vi "nanocal -- nuclear schottky fit V3.vi"() -> ()   [LabVIEW 2020] (continued)
-> 45.000000000000  |>   , \r80135 ->   <| \"ζ\"->  0.000000000000  , \"τ1\"-> 0.000000000000  , \"τS\"-> 0.000000000000  , \"τN\"-> 0.000000000000  , \"τC\"-> 0.000000000000  , \"κ0\"-> 0.000000000000  , \"mm1\"-> 0.000000000000  , \"mm2\"-> 0.000000000000  , \"mm3\"-> 0.000000000000  , \"T\"->  0.830000000000  , \"B\"-> 12.000000000000  , \"θ\"-> 45.000000000000  |>   , \r80136 ->   <| \"ζ\"->  0.000000000000  , \"τ1\"-> 0.000000000000  , \"τS\"-> 0.000000000000  , \"τN\"-> 0.000000000000  , \"τC\"-> 0.000000000000  , \"κ0\"-> 0.000000000000  , \"mm1\"-> 0.000000000000  , \"mm2\"-> 0.000000000000  , \"mm3\"-> 0.000000000000  , \"T\"->  1.130000000000  , \"B\"-> 12.000000000000  , \"θ\"-> 45.000000000000  |>   , \r80137 ->   <| \"ζ\"->  0.000000000000  , \"τ1\"-> 0.000000000000  , \"τS\"-> 0.000000000000  , \"τN\"-> 0.000000000000  , \"τC\"-> 0.000000000000  , \"κ0\"-> 0.000000000000  , \"mm1\"-> 0.000000000000  , \"mm2\"-> 0.000000000000  , \"mm3\"-> 0.000000000000  , \"T\"->  1.900000000000  , \"B\"-> 12.000000000000  , \"θ\"-> 45.000000000000  |>   , \r80138 ->   <| \"ζ\"->  0.000000000000  , \"τ1\"-> 0.000000000000  , \"τS\"-> 0.000000000000  , \"τN\"-> 0.000000000000  , \"τC\"-> 0.000000000000  , \"κ0\"-> 0.000000000000  , \"mm1\"-> 0.000000000000  , \"mm2\"-> 0.000000000000  , \"mm3\"-> 0.000000000000  , \"T\"->  3.100000000000  , \"B\"-> 12.000000000000  , \"θ\"-> 45.000000000000  |>   , \r80139 ->   <| \"ζ\"->  0.000000000000  , \"τ1\"-> 0.000000000000  , \"τS\"-> 0.000000000000  , \"τN\"-> 0.000000000000  , \"τC\"-> 0.000000000000  , \"κ0\"-> 0.000000000000  , \"mm1\"-> 0.000000000000  , \"mm2\"-> 0.000000000000  , \"mm3\"-> 0.000000000000  , \"T\"->  5.700000000000  , \"B\"-> 12.000000000000  , \"θ\"-> 45.000000000000  |>   , \r"
  out "string OUT":string="  4026 ->   <| \"ζ\"->  0.380655948508  , \"τ1\"-> 0.067955996733  , \"τS\"-> 0.077431477619  , \"τN\"-> 0.380655948508  , \"τC\"-> 0.001948284419  , \"κ0\"-> 0.000000000405  , \"mm1\"-> 0.000000000000  , \"mm2\"-> 0.000000000000  , \"mm3\"-> 0.000000000000  , \"T\"->  0.127000000000  , \"B\"-> 12.000000000000  , \"θ\"-> 60.000000000000  |>   , \r4027 ->   <| \"ζ\"->  0.301371774455  , \"τ1\"-> 0.068371484218  , \"τS\"-> 0.061790748646  , \"τN\"-> 0.216325501043  , \"τC\"-> 0.002093631430  , \"κ0\"-> 0.000000000652  , \"mm1\"-> 0.000000000000  , \"mm2\"-> 0.000000000000  , \"mm3\"-> 0.000000000000  , \"T\"->  0.150000000000  , \"B\"-> 12.000000000000  , \"θ\"-> 60.000000000000  |>   , \r4028 ->   <| \"ζ\"->  0.246466162800  , \"τ1\"-> 0.063598094006  , \"τS\"-> 0.040287819160  , \"τN\"-> 0.158425596558  , \"τC\"-> 0.002271690953  , \"κ0\"-> 0.000000000764  , \"mm1\"-> 0.000000000000  , \"mm2\"-> 0.000000000000  , \"mm3\"-> 0.000000000000  , \"T\"->  0.179000000000  , \"B\"-> 12.000000000000  , \"θ\"-> 60.000000000000  |>   , \r4029 ->   <| \"ζ\"->  0.189727451301  , \"τ1\"-> 0.058299219384  , \"τS\"-> 0.037057198532  , \"τN\"-> 0.081832461227  , \"τC\"-> 0.002345641238  , \"κ0\"-> 0.000000001055  , \"mm1\"-> 0.000000000000  , \"mm2\"-> 0.000000000000  , \"mm3\"-> 0.000000000000  , \"T\"->  0.200000000000  , \"B\"-> 12.000000000000  , \"θ\"-> 60.000000000000  |>   , \r4030 ->   <| \"ζ\"->  0.139910467625  , \"τ1\"-> 0.047050769060  , \"τS\"-> 0.031171501064  , \"τN\"-> 0.041998910400  , \"τC\"-> 0.002916001976  , \"κ0\"-> 0.000000001342  , \"mm1\"-> 0.000000000000  , \"mm2\"-> 0.000000000000  , \"mm3\"-> 0.000000000000  , \"T\"->  0.240000000000  , \"B\"-> 12.000000000000  , \"θ\"-> 60.000000000000  |>   , \r4031 ->   <| \"ζ\"->  0.099227356109  , \"τ1\"-> 0.042371773796  , \"τS\"-> 0.026407434530  , \"τN\"-> 0.023302306750  , \"τC\"-> 0.003363353135  , \"κ0\"-> 0.000000001685  , \"mm1\"-> 0.000000000000  , \"mm2\"-> 0.000000000000  , \"mm3\"-> 0.000000000000  , \"T\"->  0.287000000000  , \"B\"-> 12.000000000000  , \"θ\"-> 60.000000000000  |>   , \r4032 ->   <| \"ζ\"->  0.076929995365  , \"τ1\"-> 0.033595523097  , \"τS\"-> 0.023151959369  , \"τN\"-> 0.012952644411  , \"τC\"-> 0.004200734342  , \"κ0\"-> 0.000000002024  , \"mm1\"-> 0.000000000000  , \"mm2\"-> 0.000000000000  , \"mm3\"-> 0.000000000000  , \"T\"->  0.330000000000  , \"B\"-> 12.000000000000  , \"θ\"-> 60.000000000000  |>   , \r4033 ->   <| \"ζ\"->  0.051029693776  , \"τ1\"-> 0.027044732579  , \"τS\"-> 0.020325597844  , \"τN\"-> 0.004901643856  , \"τC\"-> 0.005324185887  , \"κ0\"-> 0.000000002659  , \"mm1\"-> 0.000000000000  , \"mm2\"-> 0.000000000000  , \"mm3\"-> 0.000000000000  , \"T\"->  0.430000000000  , \"B\"-> 12.000000000000  , \"θ\"-> 60.000000000000  |>   , \r4034 ->   <| \"ζ\"->  0.041895708972  , \"τ1\"-> 0.024266785024  , \"τS\"-> 0.017749465045  , \"τN\"-> 0.003280175510  , \"τC\"-> 0.006877927658  , \"κ0\"-> 0.000000003199  , \"mm1\"-> 0.000000000000  , \"mm2\"-> 0.000000000000  , \"mm3\"-> 0.000000000000  , \"T\"->  0.510000000000  , \"B\"-> 12.000000000000  , \"θ\"-> 60.000000000000  |>   , \r4035 ->   <| \"ζ\"->  0.038450971441  , \"τ1\"-> 0.022519642738  , \"τS\"-> 0.015666742742  , \"τN\"-> 0.001856597287  , \"τC\"-> 0.008327032616  , \"κ0\"-> 0.000000003902  , \"mm1\"-> 0.000000000000  , \"mm2\"-> 0.000000000000  , \"mm3\"-> 0.000000000000  , \"T\"->  0.620000000000  , \"B\"-> 12.000000000000  , \"θ\"-> 60.000000000000  |>   , \r4036 ->   <| \"ζ\"->  0.030292839572  , \"τ1\"-> 0.021747519944  , \"τS\"-> 0.012455692286  , \"τN\"-> 0.000770679826  , \"τC\"-> 0.010003902376  , \"κ0\"-> 0.000000005444  , \"mm1\"-> 0.000000000000  , \"mm2\"-> 0.000000000000  , \"mm3\"-> 0.000000000000  , \"T\"->  0.830000000000  , \"B\"-> 12.000000000000  , \"θ\"-> 60.000000000000  |>   , \r4037 ->   <| \"ζ\"->  0.027148872036  , \"τ1\"-> 0.019406705499  , \"τS\"-> 0.010006462721  , \"τN\"-> 0.000385841484  , \"τC\"-> 0.010479299639  , \"κ0\"-> 0.000000007587  , \"mm1\"-> 0.000000000000  , \"mm2\"-> 0.000000000000  , \"mm3\"-> 0.000000000000  , \"T\"->  1.130000000000  , \"B\"-> 12.000000000000  , \"θ\"-> 60.000000000000  |>   , \r4038 ->   <| \"ζ\"->  0.023655000000  , \"τ1\"-> 0.018908981512  , \"τS\"-> 0.006794860000  , \"τN\"-> 0.000182123000  , \"τC\"-> 0.009832330000  , \"κ0\"-> 0.000000013113  , \"mm1\"-> 0.000000000000  , \"mm2\"-> 0.000000000000  , \"mm3\"-> 0.000000000000  , \"T\"->  1.900000000000  , \"B\"-> 12.000000000000  , \"θ\"-> 60.000000000000  |>   , \r4039 ->   <| \"ζ\"->  0.020379855604  , \"τ1\"-> 0.018418482061  , \"τS\"-> 0.004575065916  , \"τN\"-> 0.000085371343  , \"τC\"-> 0.008551724457  , \"κ0\"-> 0.000000023824  , \"mm1\"-> 0.000000000000  , \"mm2\"-> 0.000000000000  , \"mm3\"-> 0.000000000000  , \"T\"->  3.150000000000  , \"B\"-> 12.000000000000  , \"θ\"-> 60.000000000000  |>   , \r4040 ->   <| \"ζ\"->  0.020744689680  , \"τ1\"-> 0.017944253087  , \"τS\"-> 0.003548154619  , \"τN\"-> 0.000036329906  , \"τC\"-> 0.004738266852  , \"κ0\"-> 0.000000058027  , \"mm1\"-> 0.000000000000  , \"mm2\"-> 0.000000000000  , \"mm3\"-> 0.000000000000  , \"T\"->  5.700000000000  , \"B\"-> 12.000000000000  , \"θ\"-> 60.000000000000  |>   , \r4041 ->   <| \"ζ\"->  0.020744689680  , \"τ1\"-> 0.017944253087  , \"τS\"-> 0.003548154619  , \"τN\"-> 0.000036329906  , \"τC\"-> 0.004738266852  , \"κ0\"-> 0.000000058027  , \"mm1\"-> 0.000000000000  , \"mm2\"-> 0.000000000000  , \"mm3\"-> 0.000000000000  , \"T\"->  7.870000000000  , \"B\"-> 12.000000000000  , \"θ\"-> 60.000000000000  |>   , \r4042 ->   <| \"ζ\"->  0.020744689680  , \"τ1\"-> 0.017944253087  , \"τS\"-> 0.003548154619  , \"τN\"-> 0.000036329906  , \"τC\"-> 0.004738266852  , \"κ0\"-> 0.000000058027  , \"mm1\"-> 0.000000000000  , \"mm2\"-> 0.000000000000  , \"mm3\"-> 0.000000000000  , \"T\"->  9.800000000000  , \"B\"-> 12.000000000000  , \"θ\"-> 60.000000000000  |>   , \r4043 ->   <| \"ζ\"->  0.020744689680  , \"τ1\"-> 0.017944253087  , \"τS\"-> 0.003548154619  , \"τN\"-> 0.000036329906  , \"τC\"-> 0.004738266852  , \"κ0\"-> 0.000000058027  , \"mm1\"-> 0.000000000000  , \"mm2\"-> 0.000000000000  , \"mm3\"-> 0.000000000000  , \"T\"->  12.360000000000  , \"B\"-> 12.000000000000  , \"θ\"-> 60.000000000000  |>   , \r4044 ->   <| \"ζ\"->  0.020744689680  , \"τ1\"-> 0.017944253087  , \"τS\"-> 0.003548154619  , \"τN\"-> 0.000036329906  , \"τC\"-> 0.004738266852  , \"κ0\"-> 0.000000058027  , \"mm1\"-> 0.000000000000  , \"mm2\"-> 0.000000000000  , \"mm3\"-> 0.000000000000  , \"T\"->  14.800000000000  , \"B\"-> 12.000000000000  , \"θ\"-> 60.000000000000  |>   , \r4045 ->   <| \"ζ\"->  0.020744689680  , \"τ1\"-> 0.017944253087  , \"τS\"-> 0.003548154619  , \"τN\"-> 0.000036329906  , \"τC\"-> 0.004738266852  , \"κ0\"-> 0.000000058027  , \"mm1\"-> 0.000000000000  , \"mm2\"-> 0.000000000000  , \"mm3\"-> 0.000000000000  , \"T\"->  16.420000000000  , \"B\"-> 12.000000000000  , \"θ\"-> 60.000000000000  |>   , \r4046 ->   <| \"ζ\"->  0.020744689680  , \"τ1\"-> 0.017944253087  , \"τS\"-> 0.003548154619  , \"τN\"-> 0.000036329906  , \"τC\"-> 0.004738266852  , \"κ0\"-> 0.000000058027  , \"mm1\"-> 0.000000000000  , \"mm2\"-> 0.000000000000  , \"mm3\"-> 0.000000000000  , \"T\"->  18.040000000000  , \"B\"-> 12.000000000000  , \"θ\"-> 60.000000000000  |>   , \r4047 ->   <| \"ζ\"->  0.300947716662  , \"τ1\"-> 0.034470276406  , \"τS\"-> 0.250683291493  , \"τN\"-> 0.334074141272  , \"τC\"-> 0.000964143340  , \"κ0\"-> 0.000000000518  , \"mm1\"-> 0.000000000000  , \"mm2\"-> 0.000000000000  , \"mm3\"-> 0.000000000000  , \"T\"->  0.140000000000  , \"B\"-> 12.000000000000  , \"θ\"-> 0.000000000000  |>   , \r4048 ->   <| \"ζ\"->  0.268000520782  , \"τ1\"-> 0.029931150536  , \"τS\"-> 0.192534253926  , \"τN\"-> 0.181611498855  , \"τC\"-> 0.001049830818  , \"κ0\"-> 0.000000000650  , \"mm1\"-> 0.000000000000  , \"mm2\"-> 0.000000000000  , \"mm3\"-> 0.000000000000  , \"T\"->  0.170000000000  , \"B\"-> 12.000000000000  , \"θ\"-> 0.000000000000  |>   , \r4049 ->   <| \"ζ\"->  0.207464615280  , \"τ1\"-> 0.027483302153  , \"τS\"-> 0.118394731157  , \"τN\"-> 0.102469315740  , \"τC\"-> 0.000943010704  , \"κ0\"-> 0.000000000915  , \"mm1\"-> 0.000000000000  , \"mm2\"-> 0.000000000000  , \"mm3\"-> 0.000000000000  , \"T\"->  0.200000000000  , \"B\"-> 12.000000000000  , \"θ\"-> 0.000000000000  |>   , \r4050 ->   <| \"ζ\"->  0.165475996734  , \"τ1\"-> 0.025963786655  , \"τS\"-> 0.093704496942  , \"τN\"-> 0.070002514088  , \"τC\"-> 0.001078811076  , \"κ0\"-> 0.000000001056  , \"mm1\"-> 0.000000000000  , \"mm2\"-> 0.000000000000  , \"mm3\"-> 0.000000000000  , \"T\"->  0.220000000000  , \"B\"-> 12.000000000000  , \"θ\"-> 0.000000000000  |>   , \r4051 ->   <| \"ζ\"->  0.095669926669  , \"τ1\"-> 0.023471442307  , \"τS\"-> 0.070780175000  , \"τN\"-> 0.023358853826  , \"τC\"-> 0.001421190467  , \"κ0\"-> 0.000000001370  , \"mm1\"-> 0.000000000000  , \"mm2\"-> 0.000000000000  , \"mm3\"-> 0.000000000000  , \"T\"->  0.280000000000  , \"B\"-> 12.000000000000  , \"θ\"-> 0.000000000000  |>   , \r4052 ->   <| \"ζ\"->  0.066045279838  , \"τ1\"-> 0.021690723483  , \"τS\"-> 0.054398710223  , \"τN\"-> 0.012159058060  , \"τC\"-> 0.001677829713  , \"κ0\"-> 0.000000001745  , \"mm1\"-> 0.000000000000  , \"mm2\"-> 0.000000000000  , \"mm3\"-> 0.000000000000  , \"T\"->  0.330000000000  , \"B\"-> 12.000000000000  , \"θ\"-> 0.000000000000  |>   , \r4053 ->   <| \"ζ\"->  0.046429657722  , \"τ1\"-> 0.021005913305  , \"τS\"-> 0.044250298502  , \"τN\"-> 0.006399419767  , \"τC\"-> 0.002349605146  , \"κ0\"-> 0.000000002166  , \"mm1\"-> 0.000000000000  , \"mm2\"-> 0.000000000000  , \"mm3\"-> 0.000000000000  , \"T\"->  0.400000000000  , \"B\"-> 12.000000000000  , \"θ\"-> 0.000000000000  |>   , \r4054 ->   <| \"ζ\"->  0.033449822896  , \"τ1\"-> 0.018946770596  , \"τS\"-> 0.035864277160  , \"τN\"-> 0.004007639534  , \"τC\"-> 0.003128970761  , \"κ0\"-> 0.000000002686  , \"mm1\"-> 0.000000000000  , \"mm2\"-> 0.000000000000  , \"mm3\"-> 0.000000000000  , \"T\"->  0.480000000000  , \"B\"-> 12.000000000000  , \"θ\"-> 0.000000000000  |>   , \r4055 ->   <| \"ζ\"->  0.026131121682  , \"τ1\"-> 0.018837612836  , \"τS\"-> 0.029051745056  , \"τN\"-> 0.002477027845  , \"τC\"-> 0.003638595201  , \"κ0\"-> 0.000000003369  , \"mm1\"-> 0.000000000000  , \"mm2\"-> 0.000000000000  , \"mm3\"-> 0.000000000000  , \"T\"->  0.580000000000  , \"B\"-> 12.000000000000  , \"θ\"-> 0.000000000000  |>   , \r4056 ->   <| \"ζ\"->  0.024432142513  , \"τ1\"-> 0.016357279945  , \"τS\"-> 0.024348527270  , \"τN\"-> 0.001658773318  , \"τC\"-> 0.004361258788  , \"κ0\"-> 0.000000003978  , \"mm1\"-> 0.000000000000  , \"mm2\"-> 0.000000000000  , \"mm3\"-> 0.000000000000  , \"T\"->  0.680000000000  , \"B\"-> 12.000000000000  , \"θ\"-> 0.000000000000  |>   , \r4057 ->   <| \"ζ\"->  0.021686886303  , \"τ1\"-> 0.014035370333  , \"τS\"-> 0.018696444406  , \"τN\"-> 0.000822758998  , \"τC\"-> 0.004334784728  , \"κ0\"-> 0.000000005544  , \"mm1\"-> 0.000000000000  , \"mm2\"-> 0.000000000000  , \"mm3\"-> 0.000000000000  , \"T\"->  0.910000000000  , \"B\"-> 12.000000000000  , \"θ\"-> 0.000000000000  |>   , \r4058 ->   <| \"ζ\"->  0.021090283514  , \"τ1\"-> 0.013945744068  , \"τS\"-> 0.014386606899  , \"τN\"-> 0.000345175874  , \"τC\"-> 0.004902956629  , \"κ0\"-> 0.000000007742  , \"mm1\"-> 0.000000000000  , \"mm2\"-> 0.000000000000  , \"mm3\"-> 0.000000000000  , \"T\"->  1.230000000000  , \"B\"-> 12.000000000000  , \"θ\"-> 0.000000000000  |>   , \r4059 ->   <| \"ζ\"->  0.021449250230  , \"τ1\"-> 0.014564522147  , \"τS\"-> 0.008878867204  , \"τN\"-> 0.000064984242  , \"τC\"-> 0.006207353748  , \"κ0\"-> 0.000000012530  , \"mm1\"-> 0.000000000000  , \"mm2\"-> 0.000000000000  , \"mm3\"-> 0.000000000000  , \"T\"->  1.970000000000  , \"B\"-> 12.000000000000  , \"θ\"-> 0.000000000000  |>   , \r4060 ->   <| \"ζ\"->  0.024633693577  , \"τ1\"-> 0.014940694735  , \"τS\"-> 0.006137734482  , \"τN\"-> 0.000014567254  , \"τC\"-> 0.005080683927  , \"κ0\"-> 0.000000022488  , \"mm1\"-> 0.000000000000  , \"mm2\"-> 0.000000000000  , \"mm3\"-> 0.000000000000  , \"T\"->  3.190000000000  , \"B\"-> 12.000000000000  , \"θ\"-> 0.000000000000  |>   , \r4061 ->   <| \"ζ\"->  0.027835388666  , \"τ1\"-> 0.013976390421  , \"τS\"-> 0.003539188638  , \"τN\"-> 0.000003774856  , \"τC\"-> 0.004420299329  , \"κ0\"-> 0.000000055482  , \"mm1\"-> 0.000000000000  , \"mm2\"-> 0.000000000000  , \"mm3\"-> 0.000000000000  , \"T\"->  5.820000000000  , \"B\"-> 12.000000000000  , \"θ\"-> 0.000000000000  |>   , \r4070 ->   <| \"ζ\"->  0.194847779603  , \"τ1\"-> 0.071300022200  , \"τS\"-> 0.034370433557  , \"τN\"-> 0.119698958932  , \"τC\"-> 0.001245041457  , \"κ0\"-> 0.000000000909  , \"mm1\"-> 0.000000000000  , \"mm2\"-> 0.000000000000  , \"mm3\"-> 0.000000000000  , \"T\"->  0.200000000000  , \"B\"-> 12.000000000000  , \"θ\"-> 90.000000000000  |>   , \r4071 ->   <| \"ζ\"->  0.269487394269  , \"τ1\"-> 0.127683064756  , \"τS\"-> 0.080630500543  , \"τN\"-> 1.047670772049  , \"τC\"-> 0.001667584944  , \"κ0\"-> 0.000000000515  , \"mm1\"-> 0.000000000000  , \"mm2\"-> 0.000000000000  , \"mm3\"-> 0.000000000000  , \"T\"->  0.140000000000  , \"B\"-> 12.000000000000  , \"θ\"-> 90.000000000000  |>   , \r4072 ->   <| \"ζ\"->  0.262382286581  , \"τ1\"-> 0.087570397050  , \"τS\"-> 0.043209451217  , \"τN\"-> 0.242360418902  , \"τC\"-> 0.001166981889  , \"κ0\"-> 0.000000000671  , \"mm1\"-> 0.000000000000  , \"mm2\"-> 0.000000000000  , \"mm3\"-> 0.000000000000  , \"T\"->  0.180000000000  , \"B\"-> 12.000000000000  , \"θ\"-> 90.000000000000  |>   , \r4073 ->   <| \"ζ\"->  0.166318035375  , \"τ1\"-> 0.066119695107  , \"τS\"-> 0.031891479777  , \"τN\"-> 0.088107606578  , \"τC\"-> 0.001299933301  , \"κ0\"-> 0.000000001075  , \"mm1\"-> 0.000000000000  , \"mm2\"-> 0.000000000000  , \"mm3\"-> 0.000000000000  , \"T\"->  0.220000000000  , \"B\"-> 12.000000000000  , \"θ\"-> 90.000000000000  |>   , \r4074 ->   <| \"ζ\"->  0.101265410351  , \"τ1\"-> 0.051590946451  , \"τS\"-> 0.026920044229  , \"τN\"-> 0.035536954174  , \"τC\"-> 0.001490330879  , \"κ0\"-> 0.000000001364  , \"mm1\"-> 0.000000000000  , \"mm2\"-> 0.000000000000  , \"mm3\"-> 0.000000000000  , \"T\"->  0.270000000000  , \"B\"-> 12.000000000000  , \"θ\"-> 90.000000000000  |>   , \r4075 ->   <| \"ζ\"->  0.070401604603  , \"τ1\"-> 0.043684283216  , \"τS\"-> 0.023756676354  , \"τN\"-> 0.017570167589  , \"τC\"-> 0.001809460237  , \"κ0\"-> 0.000000001742  , \"mm1\"-> 0.000000000000  , \"mm2\"-> 0.000000000000  , \"mm3\"-> 0.000000000000  , \"T\"->  0.330000000000  , \"B\"-> 12.000000000000  , \"θ\"-> 90.000000000000  |>   , \r4076 ->   <| \"ζ\"->  0.052039078112  , \"τ1\"-> 0.037833987996  , \"τS\"-> 0.021664376950  , \"τN\"-> 0.010364100672  , \"τC\"-> 0.002302914949  , \"κ0\"-> 0.000000002119  , \"mm1\"-> 0.000000000000  , \"mm2\"-> 0.000000000000  , \"mm3\"-> 0.000000000000  , \"T\"->  0.390000000000  , \"B\"-> 12.000000000000  , \"θ\"-> 90.000000000000  |>   , \r4077 ->   <| \"ζ\"->  0.040584680050  , \"τ1\"-> 0.030359591877  , \"τS\"-> 0.019792901852  , \"τN\"-> 0.005324821183  , \"τC\"-> 0.002700986774  , \"κ0\"-> 0.000000002671  , \"mm1\"-> 0.000000000000  , \"mm2\"-> 0.000000000000  , \"mm3\"-> 0.000000000000  , \"T\"->  0.480000000000  , \"B\"-> 12.000000000000  , \"θ\"-> 90.000000000000  |>   , \r4078 ->   <| \"ζ\"->  0.030700897923  , \"τ1\"-> 0.026935085078  , \"τS\"-> 0.018364864329  , \"τN\"-> 0.002898516959  , \"τC\"-> 0.003150649099  , \"κ0\"-> 0.000000003342  , \"mm1\"-> 0.000000000000  , \"mm2\"-> 0.000000000000  , \"mm3\"-> 0.000000000000  , \"T\"->  0.580000000000  , \"B\"-> 12.000000000000  , \"θ\"-> 90.000000000000  |>   , \r4079 ->   <| \"ζ\"->  0.025322625458  , \"τ1\"-> 0.023401812401  , \"τS\"-> 0.017347416709  , \"τN\"-> 0.002020498851  , \"τC\"-> 0.003594259467  , \"κ0\"-> 0.000000003970  , \"mm1\"-> 0.000000000000  , \"mm2\"-> 0.000000000000  , \"mm3\"-> 0.000000000000  , \"T\"->  0.680000000000  , \"B\"-> 12.000000000000  , \"θ\"-> 90.000000000000  |>   , \r4080 ->   <| \"ζ\"->  0.020909345533  , \"τ1\"-> 0.018639086414  , \"τS\"-> 0.015508870178  , \"τN\"-> 0.000897965634  , \"τC\"-> 0.004365378736  , \"κ0\"-> 0.000000005563  , \"mm1\"-> 0.000000000000  , \"mm2\"-> 0.000000000000  , \"mm3\"-> 0.000000000000  , \"T\"->  0.910000000000  , \"B\"-> 12.000000000000  , \"θ\"-> 90.000000000000  |>   , \r4081 ->   <| \"ζ\"->  0.020895919821  , \"τ1\"-> 0.022779661439  , \"τS\"-> 0.013362775673  , \"τN\"-> 0.000455286834  , \"τC\"-> 0.005327512397  , \"κ0\"-> 0.000000007772  , \"mm1\"-> 0.000000000000  , \"mm2\"-> 0.000000000000  , \"mm3\"-> 0.000000000000  , \"T\"->  1.230000000000  , \"B\"-> 12.000000000000  , \"θ\"-> 90.000000000000  |>   , \r4082 ->   <| \"ζ\"->  0.020900126456  , \"τ1\"-> 0.018293725681  , \"τS\"-> 0.009160984548  , \"τN\"-> 0.000128789786  , \"τC\"-> 0.006826962726  , \"κ0\"-> 0.000000013444  , \"mm1\"-> 0.000000000000  , \"mm2\"-> 0.000000000000  , \"mm3\"-> 0.000000000000  , \"T\"->  2.050000000000  , \"B\"-> 12.000000000000  , \"θ\"-> 90.000000000000  |>   , \r4083 ->   <| \"ζ\"->  0.019765118173  , \"τ1\"-> 0.018324978618  , \"τS\"-> 0.006054329354  , \"τN\"-> 0.000028420666  , \"τC\"-> 0.006398306925  , \"κ0\"-> 0.000000023958  , \"mm1\"-> 0.000000000000  , \"mm2\"-> 0.000000000000  , \"mm3\"-> 0.000000000000  , \"T\"->  3.310000000000  , \"B\"-> 12.000000000000  , \"θ\"-> 90.000000000000  |>   , \r4084 ->   <| \"ζ\"->  0.030164668817  , \"τ1\"-> 0.012822215558  , \"τS\"-> 0.004108197943  , \"τN\"-> 0.000006999504  , \"τC\"-> 0.004420975765  , \"κ0\"-> 0.000000058872  , \"mm1\"-> 0.000000000000  , \"mm2\"-> 0.000000000000  , \"mm3\"-> 0.000000000000  , \"T\"->  6.000000000000  , \"B\"-> 12.000000000000  , \"θ\"-> 90.000000000000  |>   , \r4094 ->   <| \"ζ\"->  0.000000000000  , \"τ1\"-> 0.000000000000  , \"τS\"-> 0.000000000000  , \"τN\"-> 0.000000000000  , \"τC\"-> 0.000000000000  , \"κ0\"-> 0.000000000000  , \"mm1\"-> 0.000000000000  , \"mm2\"-> 0.000000000000  , \"mm3\"-> 0.000000000000  , \"T\"->  0.300000000000  , \"B\"-> 6.000000000000  , \"θ\"-> 90.000000000000  |>   , \r4095 ->   <| \"ζ\"->  0.163571654798  , \"τ1\"-> 0.020520714675  , \"τS\"-> 0.073117323271  , \"τN\"-> 0.020627224399  , \"τC\"-> 0.001336341391  , \"κ0\"-> 0.000000001061  , \"mm1\"-> 0.000000000000  , \"mm2\"-> 0.000000000000  , \"mm3\"-> 0.000000000000  , \"T\"->  0.197000000000  , \"B\"-> 6.000000000000  , \"θ\"-> 90.000000000000  |>   , \r4098 ->   <| \"ζ\"->  0.000000000000  , \"τ1\"-> 0.000000000000  , \"τS\"-> 0.000000000000  , \"τN\"-> 0.000000000000  , \"τC\"-> 0.000000000000  , \"κ0\"-> 0.000000000000  , \"mm1\"-> 0.000000000000  , \"mm2\"-> 0.000000000000  , \"mm3\"-> 0.000000000000  , \"T\"->  0.148000000000  , \"B\"-> 6.000000000000  , \"θ\"-> 90.000000000000  |>   , \r4099 ->   <| \"ζ\"->  0.160882265826  , \"τ1\"-> 0.034919932965  , \"τS\"-> 0.043973777096  , \"τN\"-> 0.047289018614  , \"τC\"-> 0.001339652100  , \"κ0\"-> 0.000000001069  , \"mm1\"-> 0.000000000000  , \"mm2\"-> 0.000000000000  , \"mm3\"-> 0.000000000000  , \"T\"->  0.197000000000  , \"B\"-> 9.000000000000  , \"θ\"-> 90.000000000000  |>   , \r4100 ->   <| \"ζ\"->  0.154351103049  , \"τ1\"-> 0.051844552801  , \"τS\"-> 0.034651211615  , \"τN\"-> 0.065884588100  , \"τC\"-> 0.001166375427  , \"κ0\"-> 0.000000001084  , \"mm1\"-> 0.000000000000  , \"mm2\"-> 0.000000000000  , \"mm3\"-> 0.000000000000  , \"T\"->  0.197000000000  , \"B\"-> 11.000000000000  , \"θ\"-> 90.000000000000  |>   , \r4101 ->   <| \"ζ\"->  0.158514180755  , \"τ1\"-> 0.046388884826  , \"τS\"-> 0.038847986012  , \"τN\"-> 0.058494864948  , \"τC\"-> 0.001325817289  , \"κ0\"-> 0.000000001072  , \"mm1\"-> 0.000000000000  , \"mm2\"-> 0.000000000000  , \"mm3\"-> 0.000000000000  , \"T\"->  0.197000000000  , \"B\"-> 10.000000000000  , \"θ\"-> 90.000000000000  |>   , \r4102 ->   <| \"ζ\"->  0.154362032240  , \"τ1\"-> 0.030258273194  , \"τS\"-> 0.049523350330  , \"τN\"-> 0.040015703513  , \"τC\"-> 0.001328953616  , \"κ0\"-> 0.000000001075  , \"mm1\"-> 0.000000000000  , \"mm2\"-> 0.000000000000  , \"mm3\"-> 0.000000000000  , \"T\"->  0.197000000000  , \"B\"-> 8.000000000000  , \"θ\"-> 90.000000000000  |>   , \r4103 ->   <| \"ζ\"->  0.162645417184  , \"τ1\"-> 0.023693851446  , \"τS\"-> 0.062400062170  , \"τN\"-> 0.026326088223  , \"τC\"-> 0.001322053294  , \"κ0\"-> 0.000000001070  , \"mm1\"-> 0.000000000000  , \"mm2\"-> 0.000000000000  , \"mm3\"-> 0.000000000000  , \"T\"->  0.197000000000  , \"B\"-> 7.000000000000  , \"θ\"-> 90.000000000000  |>   , \r4104 ->   <| \"ζ\"->  0.149904026692  , \"τ1\"-> 0.020347243982  , \"τS\"-> 0.075273674904  , \"τN\"-> 0.020640082408  , \"τC\"-> 0.001432916876  , \"κ0\"-> 0.000000001050  , \"mm1\"-> 0.000000000000  , \"mm2\"-> 0.000000000000  , \"mm3\"-> 0.000000000000  , \"T\"->  0.197000000000  , \"B\"-> 5.000000000000  , \"θ\"-> 90.000000000000  |>   , \r4105 ->   <| \"ζ\"->  0.121305227705  , \"τ1\"-> 0.032098202143  , \"τS\"-> 0.011865067519  , \"τN\"-> 0.005878702730  , \"τC\"-> 0.002147559783  , \"κ0\"-> 0.000000001032  , \"mm1\"-> 0.000000000000  , \"mm2\"-> 0.000000000000  , \"mm3\"-> 0.000000000000  , \"T\"->  0.197000000000  , \"B\"-> 0.000000000000  , \"θ\"-> 90.000000000000  |>   , \r4106 ->   <| \"ζ\"->  0.000000000000  , \"τ1\"-> 0.000000000000  , \"τS\"-> 0.000000000000  , \"τN\"-> 0.000000000000  , \"τC\"-> 0.000000000000  , \"κ0\"-> 0.000000000000  , \"mm1\"-> 0.000000000000  , \"mm2\"-> 0.000000000000  , \"mm3\"-> 0.000000000000  , \"T\"->  1.550000000000  , \"B\"-> 0.000000000000  , \"θ\"-> 90.000000000000  |>   , \r4107 ->   <| \"ζ\"->  0.000000000000  , \"τ1\"-> 0.000000000000  , \"τS\"-> 0.000000000000  , \"τN\"-> 0.000000000000  , \"τC\"-> 0.000000000000  , \"κ0\"-> 0.000000000000  , \"mm1\"-> 0.000000000000  , \"mm2\"-> 0.000000000000  , \"mm3\"-> 0.000000000000  , \"T\"->  1.000000000000  , \"B\"-> 0.000000000000  , \"θ\"-> 90.000000000000  |>   , \r4108 ->   <| \"ζ\"->  0.000000000000  , \"τ1\"-> 0.000000000000  , \"τS\"-> 0.000000000000  , \"τN\"-> 0.000000000000  , \"τC\"-> 0.000000000000  , \"κ0\"-> 0.000000000000  , \"mm1\"-> 0.000000000000  , \"mm2\"-> 0.000000000000  , \"mm3\"-> 0.000000000000  , \"T\"->  0.670000000000  , \"B\"-> 0.000000000000  , \"θ\"-> 90.000000000000  |>   , \r4110 ->   <| \"ζ\"->  0.282256587364  , \"τ1\"-> 0.041594214767  , \"τS\"-> 0.086147539104  , \"τN\"-> 0.179856853536  , \"τC\"-> 0.001095910669  , \"κ0\"-> 0.000000000648  , \"mm1\"-> 0.000000000000  , \"mm2\"-> 0.000000000000  , \"mm3\"-> 0.000000000000  , \"T\"->  0.160000000000  , \"B\"-> 12.000000000000  , \"θ\"-> 30.000000000000  |>   , \r4112 ->   <| \"ζ\"->  0.271363353906  , \"τ1\"-> 0.041443755069  , \"τS\"-> 0.099499603649  , \"τN\"-> 0.147006393002  , \"τC\"-> 0.001049141338  , \"κ0\"-> 0.000000000745  , \"mm1\"-> 0.000000000000  , \"mm2\"-> 0.000000000000  , \"mm3\"-> 0.000000000000  , \"T\"->  0.170000000000  , \"B\"-> 12.000000000000  , \"θ\"-> 30.000000000000  |>   , \r4113 ->   <| \"ζ\"->  0.338385515343  , \"τ1\"-> 0.049005471612  , \"τS\"-> 0.154718584573  , \"τN\"-> 0.405362096342  , \"τC\"-> 0.001218418583  , \"κ0\"-> 0.000000000425  , \"mm1\"-> 0.000000000000  , \"mm2\"-> 0.000000000000  , \"mm3\"-> 0.000000000000  , \"T\"->  0.140000000000  , \"B\"-> 12.000000000000  , \"θ\"-> 30.000000000000  |>   , \r4114 ->   <| \"ζ\"->  0.206936374087  , \"τ1\"-> 0.035561389628  , \"τS\"-> 0.073638069843  , \"τN\"-> 0.086460784567  , \"τC\"-> 0.001118747808  , \"κ0\"-> 0.000000001040  , \"mm1\"-> 0.000000000000  , \"mm2\"-> 0.000000000000  , \"mm3\"-> 0.000000000000  , \"T\"->  0.200000000000  , \"B\"-> 12.000000000000  , \"θ\"-> 30.000000000000  |>   , \r4115 ->   <| \"ζ\"->  0.117063376722  , \"τ1\"-> 0.028106174799  , \"τS\"-> 0.053754257200  , \"τN\"-> 0.028698663234  , \"τC\"-> 0.001316309287  , \"κ0\"-> 0.000000001351  , \"mm1\"-> 0.000000000000  , \"mm2\"-> 0.000000000000  , \"mm3\"-> 0.000000000000  , \"T\"->  0.250000000000  , \"B\"-> 12.000000000000  , \"θ\"-> 30.000000000000  |>   , \r4116 ->   <| \"ζ\"->  0.083503200365  , \"τ1\"-> 0.024154552454  , \"τS\"-> 0.043596505291  , \"τN\"-> 0.014415309061  , \"τC\"-> 0.001558050220  , \"κ0\"-> 0.000000001736  , \"mm1\"-> 0.000000000000  , \"mm2\"-> 0.000000000000  , \"mm3\"-> 0.000000000000  , \"T\"->  0.300000000000  , \"B\"-> 12.000000000000  , \"θ\"-> 30.000000000000  |>   , \r4117 ->   <| \"ζ\"->  0.066204854396  , \"τ1\"-> 0.022115453498  , \"τS\"-> 0.040315193272  , \"τN\"-> 0.009107814509  , \"τC\"-> 0.001932832854  , \"κ0\"-> 0.000000002123  , \"mm1\"-> 0.000000000000  , \"mm2\"-> 0.000000000000  , \"mm3\"-> 0.000000000000  , \"T\"->  0.360000000000  , \"B\"-> 12.000000000000  , \"θ\"-> 30.000000000000  |>   , \r4118 ->   <| \"ζ\"->  0.047151602613  , \"τ1\"-> 0.020449467018  , \"τS\"-> 0.034469980201  , \"τN\"-> 0.004383898226  , \"τC\"-> 0.002055617066  , \"κ0\"-> 0.000000002642  , \"mm1\"-> 0.000000000000  , \"mm2\"-> 0.000000000000  , \"mm3\"-> 0.000000000000  , \"T\"->  0.430000000000  , \"B\"-> 12.000000000000  , \"θ\"-> 30.000000000000  |>   , \r4119 ->   <| \"ζ\"->  0.034119623194  , \"τ1\"-> 0.019653386186  , \"τS\"-> 0.029887540037  , \"τN\"-> 0.002225158248  , \"τC\"-> 0.003041304002  , \"κ0\"-> 0.000000003299  , \"mm1\"-> 0.000000000000  , \"mm2\"-> 0.000000000000  , \"mm3\"-> 0.000000000000  , \"T\"->  0.530000000000  , \"B\"-> 12.000000000000  , \"θ\"-> 30.000000000000  |>   , \r4120 ->   <| \"ζ\"->  0.027646253689  , \"τ1\"-> 0.019846033328  , \"τS\"-> 0.026627790851  , \"τN\"-> 0.001396225568  , \"τC\"-> 0.003492513642  , \"κ0\"-> 0.000000003909  , \"mm1\"-> 0.000000000000  , \"mm2\"-> 0.000000000000  , \"mm3\"-> 0.000000000000  , \"T\"->  0.620000000000  , \"B\"-> 12.000000000000  , \"θ\"-> 30.000000000000  |>   , \r4121 ->   <| \"ζ\"->  0.021289486927  , \"τ1\"-> 0.020280543944  , \"τS\"-> 0.021209329853  , \"τN\"-> 0.000861491542  , \"τC\"-> 0.004079950225  , \"κ0\"-> 0.000000005431  , \"mm1\"-> 0.000000000000  , \"mm2\"-> 0.000000000000  , \"mm3\"-> 0.000000000000  , \"T\"->  0.830000000000  , \"B\"-> 12.000000000000  , \"θ\"-> 30.000000000000  |>   , \r4122 ->   <| \"ζ\"->  0.017438026946  , \"τ1\"-> 0.020462647610  , \"τS\"-> 0.016753258897  , \"τN\"-> 0.000520420479  , \"τC\"-> 0.004207921766  , \"κ0\"-> 0.000000007613  , \"mm1\"-> 0.000000000000  , \"mm2\"-> 0.000000000000  , \"mm3\"-> 0.000000000000  , \"T\"->  1.130000000000  , \"B\"-> 12.000000000000  , \"θ\"-> 30.000000000000  |>   , \r4123 ->   <| \"ζ\"->  0.016024491492  , \"τ1\"-> 0.020653048802  , \"τS\"-> 0.011065599363  , \"τN\"-> 0.000170904127  , \"τC\"-> 0.004501051440  , \"κ0\"-> 0.000000013123  , \"mm1\"-> 0.000000000000  , \"mm2\"-> 0.000000000000  , \"mm3\"-> 0.000000000000  , \"T\"->  1.900000000000  , \"B\"-> 12.000000000000  , \"θ\"-> 30.000000000000  |>   , \r4124 ->   <| \"ζ\"->  0.018571356814  , \"τ1\"-> 0.020537072361  , \"τS\"-> 0.007110096223  , \"τN\"-> 0.000081792866  , \"τC\"-> 0.004406299379  , \"κ0\"-> 0.000000023512  , \"mm1\"-> 0.000000000000  , \"mm2\"-> 0.000000000000  , \"mm3\"-> 0.000000000000  , \"T\"->  3.100000000000  , \"B\"-> 12.000000000000  , \"θ\"-> 30.000000000000  |>   , \r8026 ->   <| \"ζ\"->  0.226997000000  , \"τ1\"-> 0.061001000000  , \"τS\"-> 0.056065000000  , \"τN\"-> 0.451284000000  , \"τC\"-> 0.001917000000  , \"κ0\"-> 0.000000000541  , \"mm1\"-> 0.000000000000  , \"mm2\"-> 0.000000000000  , \"mm3\"-> 0.000000000000  , \"T\"->  0.127000000000  , \"B\"-> 12.000000000000  , \"θ\"-> 60.000000000000  |>   , \r8027 ->   <| \"ζ\"->  0.172926301574  , \"τ1\"-> 0.059570486348  , \"τS\"-> 0.050344582002  , \"τN\"-> 0.265837950917  , \"τC\"-> 0.001945823967  , \"κ0\"-> 0.000000000779  , \"mm1\"-> 0.000000000000  , \"mm2\"-> 0.000000000000  , \"mm3\"-> 0.000000000000  , \"T\"->  0.150000000000  , \"B\"-> 12.000000000000  , \"θ\"-> 60.000000000000  |>   , \r8028 ->   <| \"ζ\"->  0.148902664674  , \"τ1\"-> 0.053249092192  , \"τS\"-> 0.052262765310  , \"τN\"-> 0.169789454991  , \"τC\"-> 0.002259759037  , \"κ0\"-> 0.000000000876  , \"mm1\"-> 0.000000000000  , \"mm2\"-> 0.000000000000  , \"mm3\"-> 0.000000000000  , \"T\"->  0.179000000000  , \"B\"-> 12.000000000000  , \"θ\"-> 60.000000000000  |>   , \r8029 ->   <| \"ζ\"->  0.112487722964  , \"τ1\"-> 0.051395902330  , \"τS\"-> 0.046676654477  , \"τN\"-> 0.101658461283  , \"τC\"-> 0.002724334068  , \"κ0\"-> 0.000000001186  , \"mm1\"-> 0.000000000000  , \"mm2\"-> 0.000000000000  , \"mm3\"-> 0.000000000000  , \"T\"->  0.200000000000  , \"B\"-> 12.000000000000  , \"θ\"-> 60.000000000000  |>   , \r8030 ->   <| \"ζ\"->  0.086003233788  , \"τ1\"-> 0.048496801153  , \"τS\"-> 0.044168635092  , \"τN\"-> 0.056305790348  , \"τC\"-> 0.004231546790  , \"κ0\"-> 0.000000001462  , \"mm1\"-> 0.000000000000  , \"mm2\"-> 0.000000000000  , \"mm3\"-> 0.000000000000  , \"T\"->  0.240000000000  , \"B\"-> 12.000000000000  , \"θ\"-> 60.000000000000  |>   , \r8031 ->   <| \"ζ\"->  0.057384090127  , \"τ1\"-> 0.040985919910  , \"τS\"-> 0.035958032989  , \"τN\"-> 0.030082348419  , \"τC\"-> 0.004188092728  , \"κ0\"-> 0.000000001825  , \"mm1\"-> 0.000000000000  , \"mm2\"-> 0.000000000000  , \"mm3\"-> 0.000000000000  , \"T\"->  0.287000000000  , \"B\"-> 12.000000000000  , \"θ\"-> 60.000000000000  |>   , \r8032 ->   <| \"ζ\"->  0.043350504485  , \"τ1\"-> 0.035291986431  , \"τS\"-> 0.032748907144  , \"τN\"-> 0.017241468603  , \"τC\"-> 0.005241482788  , \"κ0\"-> 0.000000002152  , \"mm1\"-> 0.000000000000  , \"mm2\"-> 0.000000000000  , \"mm3\"-> 0.000000000000  , \"T\"->  0.330000000000  , \"B\"-> 12.000000000000  , \"θ\"-> 60.000000000000  |>   , \r8033 ->   <| \"ζ\"->  0.024739987039  , \"τ1\"-> 0.030389077736  , \"τS\"-> 0.031546934636  , \"τN\"-> 0.007979884290  , \"τC\"-> 0.005340402456  , \"κ0\"-> 0.000000002860  , \"mm1\"-> 0.000000000000  , \"mm2\"-> 0.000000000000  , \"mm3\"-> 0.000000000000  , \"T\"->  0.430000000000  , \"B\"-> 12.000000000000  , \"θ\"-> 60.000000000000  |>   , \r8034 ->   <| \"ζ\"->  0.017670248411  , \"τ1\"-> 0.029826184303  , \"τS\"-> 0.029273717282  , \"τN\"-> 0.004773699195  , \"τC\"-> 0.006202011547  , \"κ0\"-> 0.000000003450  , \"mm1\"-> 0.000000000000  , \"mm2\"-> 0.000000000000  , \"mm3\"-> 0.000000000000  , \"T\"->  0.510000000000  , \"B\"-> 12.000000000000  , \"θ\"-> 60.000000000000  |>   , \r8035 ->   <| \"ζ\"->  0.013857502217  , \"τ1\"-> 0.024739987039  , \"τS\"-> 0.022532031675  , \"τN\"-> 0.002673871537  , \"τC\"-> 0.006319058754  , \"κ0\"-> 0.000000004207  , \"mm1\"-> 0.000000000000  , \"mm2\"-> 0.000000000000  , \"mm3\"-> 0.000000000000  , \"T\"->  0.620000000000  , \"B\"-> 12.000000000000  , \"θ\"-> 60.000000000000  |>   , \r8036 ->   <| \"ζ\"->  0.008522550050  , \"τ1\"-> 0.024739987039  , \"τS\"-> 0.016706411949  , \"τN\"-> 0.001416010776  , \"τC\"-> 0.006938274982  , \"κ0\"-> 0.000000005839  , \"mm1\"-> 0.000000000000  , \"mm2\"-> 0.000000000000  , \"mm3\"-> 0.000000000000  , \"T\"->  0.830000000000  , \"B\"-> 12.000000000000  , \"θ\"-> 60.000000000000  |>   , \r8037 ->   <| \"ζ\"->  0.005755105359  , \"τ1\"-> 0.019922509440  , \"τS\"-> 0.014656977648  , \"τN\"-> 0.000670306824  , \"τC\"-> 0.007908429886  , \"κ0\"-> 0.000000008190  , \"mm1\"-> 0.000000000000  , \"mm2\"-> 0.000000000000  , \"mm3\"-> 0.000000000000  , \"T\"->  1.130000000000  , \"B\"-> 12.000000000000  , \"θ\"-> 60.000000000000  |>   , \r8038 ->   <| \"ζ\"->  0.003814320430  , \"τ1\"-> 0.018421720348  , \"τS\"-> 0.011291290594  , \"τN\"-> 0.000268276083  , \"τC\"-> 0.009845081970  , \"κ0\"-> 0.000000013900  , \"mm1\"-> 0.000000000000  , \"mm2\"-> 0.000000000000  , \"mm3\"-> 0.000000000000  , \"T\"->  1.900000000000  , \"B\"-> 12.000000000000  , \"θ\"-> 60.000000000000  |>   , \r8039 ->   <| \"ζ\"->  0.003101094202  , \"τ1\"-> 0.017947015305  , \"τS\"-> 0.009344228121  , \"τN\"-> 0.000104308237  , \"τC\"-> 0.008562742610  , \"κ0\"-> 0.000000024300  , \"mm1\"-> 0.000000000000  , \"mm2\"-> 0.000000000000  , \"mm3\"-> 0.000000000000  , \"T\"->  3.150000000000  , \"B\"-> 12.000000000000  , \"θ\"-> 60.000000000000  |>   , \r8040 ->   <| \"ζ\"->  0.002739426716  , \"τ1\"-> 0.017947015305  , \"τS\"-> 0.006831058554  , \"τN\"-> 0.000031540596  , \"τC\"-> 0.006316465842  , \"κ0\"-> 0.000000059000  , \"mm1\"-> 0.000000000000  , \"mm2\"-> 0.000000000000  , \"mm3\"-> 0.000000000000  , \"T\"->  5.700000000000  , \"B\"-> 12.000000000000  , \"θ\"-> 60.000000000000  |>   , \r8041 ->   <| \"ζ\"->  0.000000000000  , \"τ1\"-> 0.000000000000  , \"τS\"-> 0.000000000000  , \"τN\"-> 0.000000000000  , \"τC\"-> 0.000000000000  , \"κ0\"-> 0.000000000000  , \"mm1\"-> 0.000000000000  , \"mm2\"-> 0.000000000000  , \"mm3\"-> 0.000000000000  , \"T\"->  7.870000000000  , \"B\"-> 12.000000000000  , \"θ\"-> 60.000000000000  |>   , \r8042 ->   <| \"ζ\"->  0.000000000000  , \"τ1\"-> 0.000000000000  , \"τS\"-> 0.000000000000  , \"τN\"-> 0.000000000000  , \"τC\"-> 0.000000000000  , \"κ0\"-> 0.000000000000  , \"mm1\"-> 0.000000000000  , \"mm2\"-> 0.000000000000  , \"mm3\"-> 0.000000000000  , \"T\"->  9.800000000000  , \"B\"-> 12.000000000000  , \"θ\"-> 60.000000000000  |>   , \r8043 ->   <| \"ζ\"->  0.000000000000  , \"τ1\"-> 0.000000000000  , \"τS\"-> 0.000000000000  , \"τN\"-> 0.000000000000  , \"τC\"-> 0.000000000000  , \"κ0\"-> 0.000000000000  , \"mm1\"-> 0.000000000000  , \"mm2\"-> 0.000000000000  , \"mm3\"-> 0.000000000000  , \"T\"->  12.360000000000  , \"B\"-> 12.000000000000  , \"θ\"-> 60.000000000000  |>   , \r8044 ->   <| \"ζ\"->  0.000000000000  , \"τ1\"-> 0.000000000000  , \"τS\"-> 0.000000000000  , \"τN\"-> 0.000000000000  , \"τC\"-> 0.000000000000  , \"κ0\"-> 0.000000000000  , \"mm1\"-> 0.000000000000  , \"mm2\"-> 0.000000000000  , \"mm3\"-> 0.000000000000  , \"T\"->  14.800000000000  , \"B\"-> 12.000000000000  , \"θ\"-> 60.000000000000  |>   , \r8045 ->   <| \"ζ\"->  0.000000000000  , \"τ1\"-> 0.000000000000  , \"τS\"-> 0.000000000000  , \"τN\"-> 0.000000000000  , \"τC\"-> 0.000000000000  , \"κ0\"-> 0.000000000000  , \"mm1\"-> 0.000000000000  , \"mm2\"-> 0.000000000000  , \"mm3\"-> 0.000000000000  , \"T\"->  16.420000000000  , \"B\"-> 12.000000000000  , \"θ\"-> 60.000000000000  |>   , \r8046 ->   <| \"ζ\"->  0.000000000000  , \"τ1\"-> 0.000000000000  , \"τS\"-> 0.000000000000  , \"τN\"-> 0.000000000000  , \"τC\"-> 0.000000000000  , \"κ0\"-> 0.000000000000  , \"mm1\"-> 0.000000000000  , \"mm2\"-> 0.000000000000  , \"mm3\"-> 0.000000000000  , \"T\"->  18.040000000000  , \"B\"-> 12.000000000000  , \"θ\"-> 60.000000000000  |>   , \r8047 ->   <| \"ζ\"->  0.286336668596  , \"τ1\"-> 0.037477267671  , \"τS\"-> 0.354459287884  , \"τN\"-> 0.444916383639  , \"τC\"-> 0.001225600579  , \"κ0\"-> 0.000000000596  , \"mm1\"-> 0.000000000000  , \"mm2\"-> 0.000000000000  , \"mm3\"-> 0.000000000000  , \"T\"->  0.120000000000  , \"B\"-> 12.000000000000  , \"θ\"-> 0.000000000000  |>   , \r8048 ->   <| \"ζ\"->  0.219100303741  , \"τ1\"-> 0.028643012604  , \"τS\"-> 0.279362928811  , \"τN\"-> 0.246156444058  , \"τC\"-> 0.001272401549  , \"κ0\"-> 0.000000000760  , \"mm1\"-> 0.000000000000  , \"mm2\"-> 0.000000000000  , \"mm3\"-> 0.000000000000  , \"T\"->  0.148000000000  , \"B\"-> 12.000000000000  , \"θ\"-> 0.000000000000  |>   , \r8049 ->   <| \"ζ\"->  0.170488637524  , \"τ1\"-> 0.029234231120  , \"τS\"-> 0.149095458227  , \"τN\"-> 0.151792620275  , \"τC\"-> 0.001113424175  , \"κ0\"-> 0.000000001042  , \"mm1\"-> 0.000000000000  , \"mm2\"-> 0.000000000000  , \"mm3\"-> 0.000000000000  , \"T\"->  0.179000000000  , \"B\"-> 12.000000000000  , \"θ\"-> 0.000000000000  |>   , \r8050 ->   <| \"ζ\"->  0.130531197151  , \"τ1\"-> 0.025704482770  , \"τS\"-> 0.129606657196  , \"τN\"-> 0.091602369165  , \"τC\"-> 0.001441379995  , \"κ0\"-> 0.000000001211  , \"mm1\"-> 0.000000000000  , \"mm2\"-> 0.000000000000  , \"mm3\"-> 0.000000000000  , \"T\"->  0.197000000000  , \"B\"-> 12.000000000000  , \"θ\"-> 0.000000000000  |>   , \r8051 ->   <| \"ζ\"->  0.078258046754  , \"τ1\"-> 0.028009840731  , \"τS\"-> 0.092122038762  , \"τN\"-> 0.030129595899  , \"τC\"-> 0.001641062244  , \"κ0\"-> 0.000000001543  , \"mm1\"-> 0.000000000000  , \"mm2\"-> 0.000000000000  , \"mm3\"-> 0.000000000000  , \"T\"->  0.250000000000  , \"B\"-> 12.000000000000  , \"θ\"-> 0.000000000000  |>   , \r8052 ->   <| \"ζ\"->  0.054088186012  , \"τ1\"-> 0.023838802615  , \"τS\"-> 0.069079396629  , \"τN\"-> 0.016435267456  , \"τC\"-> 0.002025071743  , \"κ0\"-> 0.000000001955  , \"mm1\"-> 0.000000000000  , \"mm2\"-> 0.000000000000  , \"mm3\"-> 0.000000000000  , \"T\"->  0.300000000000  , \"B\"-> 12.000000000000  , \"θ\"-> 0.000000000000  |>   , \r8053 ->   <| \"ζ\"->  0.039314966212  , \"τ1\"-> 0.020712803909  , \"τS\"-> 0.055413767550  , \"τN\"-> 0.008474403424  , \"τC\"-> 0.002674063387  , \"κ0\"-> 0.000000002415  , \"mm1\"-> 0.000000000000  , \"mm2\"-> 0.000000000000  , \"mm3\"-> 0.000000000000  , \"T\"->  0.360000000000  , \"B\"-> 12.000000000000  , \"θ\"-> 0.000000000000  |>   , \r8054 ->   <| \"ζ\"->  0.031945976845  , \"τ1\"-> 0.019000922826  , \"τS\"-> 0.045624146388  , \"τN\"-> 0.005314716063  , \"τC\"-> 0.002488383471  , \"κ0\"-> 0.000000002954  , \"mm1\"-> 0.000000000000  , \"mm2\"-> 0.000000000000  , \"mm3\"-> 0.000000000000  , \"T\"->  0.430000000000  , \"B\"-> 12.000000000000  , \"θ\"-> 0.000000000000  |>   , \r8055 ->   <| \"ζ\"->  0.023031239946  , \"τ1\"-> 0.018268814012  , \"τS\"-> 0.037269400776  , \"τN\"-> 0.002696792890  , \"τC\"-> 0.003257395394  , \"κ0\"-> 0.000000003720  , \"mm1\"-> 0.000000000000  , \"mm2\"-> 0.000000000000  , \"mm3\"-> 0.000000000000  , \"T\"->  0.512000000000  , \"B\"-> 12.000000000000  , \"θ\"-> 0.000000000000  |>   , \r8056 ->   <| \"ζ\"->  0.019920170845  , \"τ1\"-> 0.016368892412  , \"τS\"-> 0.030579536580  , \"τN\"-> 0.001736017565  , \"τC\"-> 0.004971418152  , \"κ0\"-> 0.000000004410  , \"mm1\"-> 0.000000000000  , \"mm2\"-> 0.000000000000  , \"mm3\"-> 0.000000000000  , \"T\"->  0.610000000000  , \"B\"-> 12.000000000000  , \"θ\"-> 0.000000000000  |>   , \r8057 ->   <| \"ζ\"->  0.017558473054  , \"τ1\"-> 0.014545104284  , \"τS\"-> 0.022979681288  , \"τN\"-> 0.000840829385  , \"τC\"-> 0.005228030240  , \"κ0\"-> 0.000000006068  , \"mm1\"-> 0.000000000000  , \"mm2\"-> 0.000000000000  , \"mm3\"-> 0.000000000000  , \"T\"->  0.810000000000  , \"B\"-> 12.000000000000  , \"θ\"-> 0.000000000000  |>   , \r8058 ->   <| \"ζ\"->  0.011916480594  , \"τ1\"-> 0.012551282481  , \"τS\"-> 0.018233218660  , \"τN\"-> 0.000345702746  , \"τC\"-> 0.004699451527  , \"κ0\"-> 0.000000008451  , \"mm1\"-> 0.000000000000  , \"mm2\"-> 0.000000000000  , \"mm3\"-> 0.000000000000  , \"T\"->  1.120000000000  , \"B\"-> 12.000000000000  , \"θ\"-> 0.000000000000  |>   , \r8059 ->   <| \"ζ\"->  0.012831327568  , \"τ1\"-> 0.013315909415  , \"τS\"-> 0.012590836847  , \"τN\"-> 0.000065003013  , \"τC\"-> 0.005276356243  , \"κ0\"-> 0.000000013610  , \"mm1\"-> 0.000000000000  , \"mm2\"-> 0.000000000000  , \"mm3\"-> 0.000000000000  , \"T\"->  1.800000000000  , \"B\"-> 12.000000000000  , \"θ\"-> 0.000000000000  |>   , \r8060 ->   <| \"ζ\"->  0.019774146838  , \"τ1\"-> 0.013257273421  , \"τS\"-> 0.007064131508  , \"τN\"-> 0.000028000819  , \"τC\"-> 0.006942241845  , \"κ0\"-> 0.000000023477  , \"mm1\"-> 0.000000000000  , \"mm2\"-> 0.000000000000  , \"mm3\"-> 0.000000000000  , \"T\"->  3.000000000000  , \"B\"-> 12.000000000000  , \"θ\"-> 0.000000000000  |>   , \r8061 ->   <| \"ζ\"->  0.029251354442  , \"τ1\"-> 0.014634751206  , \"τS\"-> 0.003873958746  , \"τN\"-> 0.000007000487  , \"τC\"-> 0.006827504775  , \"κ0\"-> 0.000000056438  , \"mm1\"-> 0.000000000000  , \"mm2\"-> 0.000000000000  , \"mm3\"-> 0.000000000000  , \"T\"->  5.500000000000  , \"B\"-> 12.000000000000  , \"θ\"-> 0.000000000000  |>   , \r8070 ->   <| \"ζ\"->  0.161975781729  , \"τ1\"-> 0.073089805113  , \"τS\"-> 0.045018408115  , \"τN\"-> 0.161987434028  , \"τC\"-> 0.001482104484  , \"κ0\"-> 0.000000001038  , \"mm1\"-> 0.000000000000  , \"mm2\"-> 0.000000000000  , \"mm3\"-> 0.000000000000  , \"T\"->  0.179000000000  , \"B\"-> 12.000000000000  , \"θ\"-> 90.000000000000  |>   , \r8071 ->   <| \"ζ\"->  0.300863384227  , \"τ1\"-> 0.104924004009  , \"τS\"-> 0.071070599729  , \"τN\"-> 0.992887187112  , \"τC\"-> 0.001721587800  , \"κ0\"-> 0.000000000548  , \"mm1\"-> 0.000000000000  , \"mm2\"-> 0.000000000000  , \"mm3\"-> 0.000000000000  , \"T\"->  0.120000000000  , \"B\"-> 12.000000000000  , \"θ\"-> 90.000000000000  |>   , \r8072 ->   <| \"ζ\"->  0.215697702358  , \"τ1\"-> 0.095971807771  , \"τS\"-> 0.069319630290  , \"τN\"-> 0.366712218878  , \"τC\"-> 0.001526252261  , \"κ0\"-> 0.000000000784  , \"mm1\"-> 0.000000000000  , \"mm2\"-> 0.000000000000  , \"mm3\"-> 0.000000000000  , \"T\"->  0.148000000000  , \"B\"-> 12.000000000000  , \"θ\"-> 90.000000000000  |>   , \r8073 ->   <| \"ζ\"->  0.139117463690  , \"τ1\"-> 0.070330410174  , \"τS\"-> 0.040829719954  , \"τN\"-> 0.122434321115  , \"τC\"-> 0.001436112939  , \"κ0\"-> 0.000000001208  , \"mm1\"-> 0.000000000000  , \"mm2\"-> 0.000000000000  , \"mm3\"-> 0.000000000000  , \"T\"->  0.197000000000  , \"B\"-> 12.000000000000  , \"θ\"-> 90.000000000000  |>   , \r8074 ->   <| \"ζ\"->  0.079912790251  , \"τ1\"-> 0.053932962768  , \"τS\"-> 0.033847624645  , \"τN\"-> 0.047947649984  , \"τC\"-> 0.001828917906  , \"κ0\"-> 0.000000001546  , \"mm1\"-> 0.000000000000  , \"mm2\"-> 0.000000000000  , \"mm3\"-> 0.000000000000  , \"T\"->  0.249000000000  , \"B\"-> 12.000000000000  , \"θ\"-> 90.000000000000  |>   , \r8075 ->   <| \"ζ\"->  0.057938569833  , \"τ1\"-> 0.045244527663  , \"τS\"-> 0.029709028064  , \"τN\"-> 0.023577376257  , \"τC\"-> 0.002006607539  , \"κ0\"-> 0.000000001948  , \"mm1\"-> 0.000000000000  , \"mm2\"-> 0.000000000000  , \"mm3\"-> 0.000000000000  , \"T\"->  0.300000000000  , \"B\"-> 12.000000000000  , \"θ\"-> 90.000000000000  |>   , \r8076 ->   <| \"ζ\"->  0.044154556051  , \"τ1\"-> 0.038823125235  , \"τS\"-> 0.027069314930  , \"τN\"-> 0.013601990730  , \"τC\"-> 0.002287979276  , \"κ0\"-> 0.000000002359  , \"mm1\"-> 0.000000000000  , \"mm2\"-> 0.000000000000  , \"mm3\"-> 0.000000000000  , \"T\"->  0.360000000000  , \"B\"-> 12.000000000000  , \"θ\"-> 90.000000000000  |>   , \r8077 ->   <| \"ζ\"->  0.032748569996  , \"τ1\"-> 0.031072007290  , \"τS\"-> 0.024343937548  , \"τN\"-> 0.006961654481  , \"τC\"-> 0.002967111565  , \"κ0\"-> 0.000000002964  , \"mm1\"-> 0.000000000000  , \"mm2\"-> 0.000000000000  , \"mm3\"-> 0.000000000000  , \"T\"->  0.430000000000  , \"B\"-> 12.000000000000  , \"θ\"-> 90.000000000000  |>   , \r8078 ->   <| \"ζ\"->  0.027599263457  , \"τ1\"-> 0.026239105728  , \"τS\"-> 0.022370859308  , \"τN\"-> 0.003857632966  , \"τC\"-> 0.003499360499  , \"
